vi "GraphWrite2File 4.vi"(6 "Calling VIs path":path, 7 "Save the Graph":bool, 8 "Comments to go in Header":string, 9 "Graph to be Saved":cluster{"Time":dbl[], "Peak-bkg Value":dbl[]}(graph), 10 "ProjectName":string="QFinger", 11 "Folder path input":path=path "C:/Labview34970A stuff/Data") -> (1 "Column Names":string[](array[string])=["Xname", "Yname"], 2 "Header":string, 3 "new file path that was created":path)   [LabVIEW 2012]
doc: "This takes a graph as input and writes it to a file. It grabs the column labels from the graph display.\nThe file naming is automated with DataFileCreator.vi\nDataFileCreator.vi is given an input Folder path and ProjectName this VI creates the next data file in the format \n2017-09-17ProjectName#001\nIt only checks the latest file in the folder to decide if \na sequence with today's date already exists.\nIf the file sequence has not been started, it creates one begining with #001\nIf it happens that it tries to create a file that already exists, a dialog pops up\nasking for a new name.\nAdd any comments you want saved in the file.\nPush the \"Save the Graph\" if you want the save to happen. This eliminates the need for the query in the main program."
uses:
  <vilib>/Utility/file.llb/Write To Spreadsheet File (DBL).vi
panel:
  # "This takes a graph as input and writes it to a file. It grabs the column labels from the graph display.\nThe file naming is automated with DataFileCreator.vi\nDataFileCreator.vi is given an input Folder path and ProjectName this VI creates the next data file in the format \n2017-09-17ProjectName#001\nIt only checks the latest file in the folder to decide if \na sequence with today's date already exists.\nIf the file sequence has not been started, it creates one begining with #001\nIf it happens that it tries to create a file that already exists, a dialog pops up\nasking for a new name.\nAdd any comments you want saved in the file.\nPush the \"Save the Graph\" if you want the save to happen. This eliminates the need for the query in the main program."
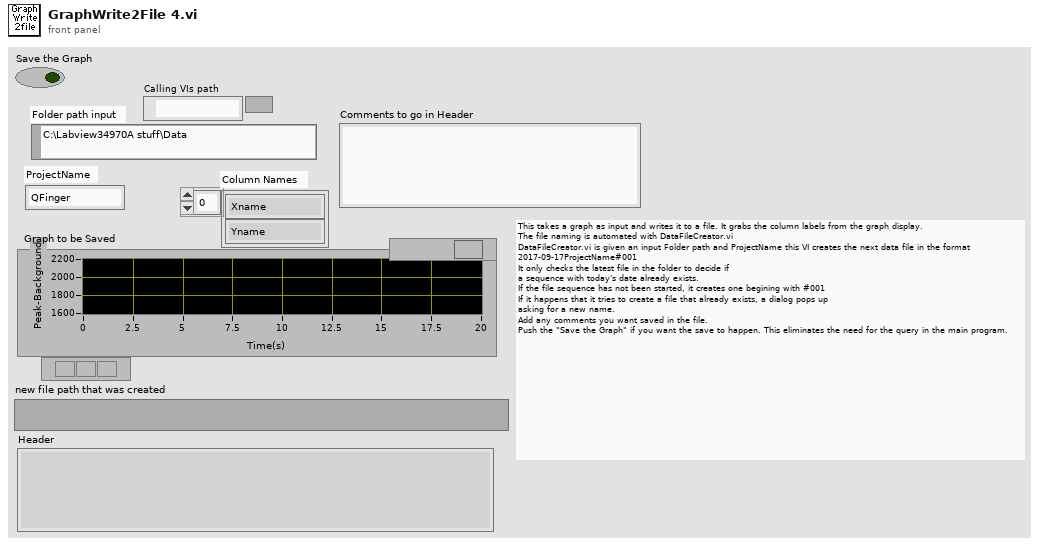
[diagram p1: front panel]
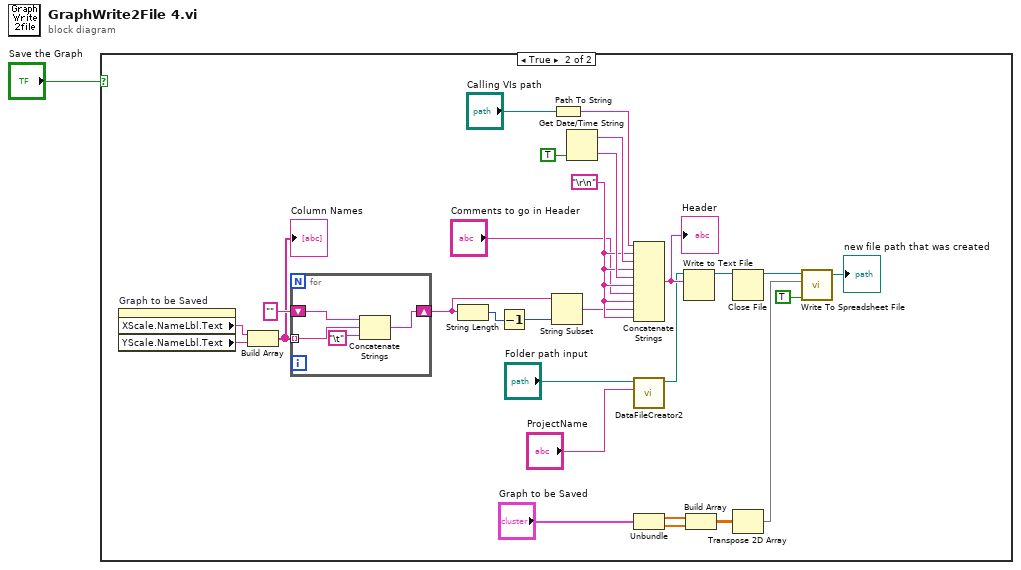
[diagram p0: block diagram]
diagram:
  n1 = case shown="True" "Save the Graph" {
    frame False {
    }
    frame True {
      w11 = "\r\n"
      n2 = property on="Graph to be Saved" class="XYGraph (strict)"() -> ("XScale.NameLbl.Text"=w5:string, "YScale.NameLbl.Text"=w4:string)  [unwired: 2 in, 2 out]
      n3 = Build Array(w5, w4) -> (w3:string[])
      "Column Names" <- w3
      n4 = for {
        shift-right: [w32] -> w23
        shift-left: "" -> [w33]
        tunnel: w3 -> [w30] mode=indexing
        n5 = Concatenate Strings(w33, w30, "\t") -> (w32:string)
      }
      n6 = String Length(string=w23) -> (length=w22:i32)
      n7 = Decrement(x=w22) -> (x-1=w21:i32)
      n8 = String Subset(string=w23, length (rest)=w21) -> (substring=w10:string)  [unwired: 1 in]
      n9 = Path To String(path="Calling VIs path") -> (string=w28:string)
      n10 = Get Date/Time String(want seconds? (F)=TRUE) -> (date string=w27:string, time string=w26:string)  [unwired: 2 in]
      n11 = Concatenate Strings(w28, w11, w27, w11, w26, w11, "Comments to go in Header", w11, w10, w11) -> (w25:string)
      "Header" <- w25
      n12 = call "DataFileCreator2.vi"("ProjectName"="ProjectName", "Folder path input"="Folder path input") -> ("NewFilePath"=w15:path)  [unwired: 8 in, 1 out]
      n13 = Unbundle("Graph to be Saved") -> ("Time"=w7:dbl[], "Peak-bkg Value"=w6:dbl[])
      n14 = Write to Text File(file (use dialog)=w15, text=w25) -> (refnum out=w14:refnum<file>)  [unwired: 2 in, 2 out]
      n15 = Build Array(w7, w6) -> (w29:dbl[][])
      n16 = Close File(refnum=w14) -> (path=w13:path)  [unwired: 1 in, 1 out]
      n17 = Transpose 2D Array(2D array=w29) -> (transposed array=w24:dbl[][])
      n18 = call-poly <vilib>:"Write To Spreadsheet File.vi"("append to file? (new file:F)"=TRUE, "2D data"=w24, "file path (dialog if empty)"=w13) -> ("new file path (Not A Path if cancelled)"=→"new file path that was created":path)  [unwired: 5 in]
    }
  }
